vi "uTTA_Calibration_Curr.vi"(6 "AR488_In":refnum<visa-resource-name>, 7 "CommandQueue":refnum<queue>, 8 "error in":errorcluster, 9 "FunctionGen_In":refnum<visa-resource-name>, 10 "DataQueue":refnum<queue>, 11 "TDMS_FileIn":refnum<k34>) -> (0 "error out":errorcluster, 1 "FunctionGen_Out":refnum<visa-resource-name>, 3 "TDMS_FileOut":refnum<k34>, 4 "AR488_Out":refnum<visa-resource-name>)   [LabVIEW 2021]
uses:
  <vilib>/Utility/miscctls.llb/LVPointTypeDef.ctl
  <vilib>/Analysis/6fits.llb/Curve Fitting Criteria.ctl
  <vilib>/Analysis/NI_AALPro.lvlib
panel:
  out "ADC offset":dbl format="%#_6pA"
  out "ADC lin. res":dbl caption="Residue" format="%.3p"
  out "ADC slope":dbl format="%#_4pA/Digit"
  out "ADC_Variance":dbl[](array[numeric]) format="%#.2g"
  out "ADC_Values":dbl[](array[numeric]) format="%#.2g"
  out "Curr ADC Cal.":cluster{"X":dbl, "Y":dbl}[](graph)
  in  "Get Measurement":bool
  in  "Shunt Resistance":dbl=0.00375 format="%#_3pOhm"
  out "Total Measurements":u32
  in  "Complete Cal":bool
  out "Status":string="Exit"
  in  "abort":bool
  # "1. Connect a power supply through a low resistance value shunt ( 10-100mOhm) to the JUT Current Input (J107) of uTTA.\n2. Connect the ground of the power supply to J106 of uTTA.\n3. Connect the sense leads of your multimeter to the sense terminals of the shunt.\n4. Set the power supply to a low current setting (~100mA).\n5. Get a measurement\n6. Set a higher current to the power supply. Steps of 1A to 2A should be sufficient.\n7. Repeat steps 5 and 6 multiple times until you have a good number of measurements.\n8. To finalize the calibration press \"Complete Calibration\"."
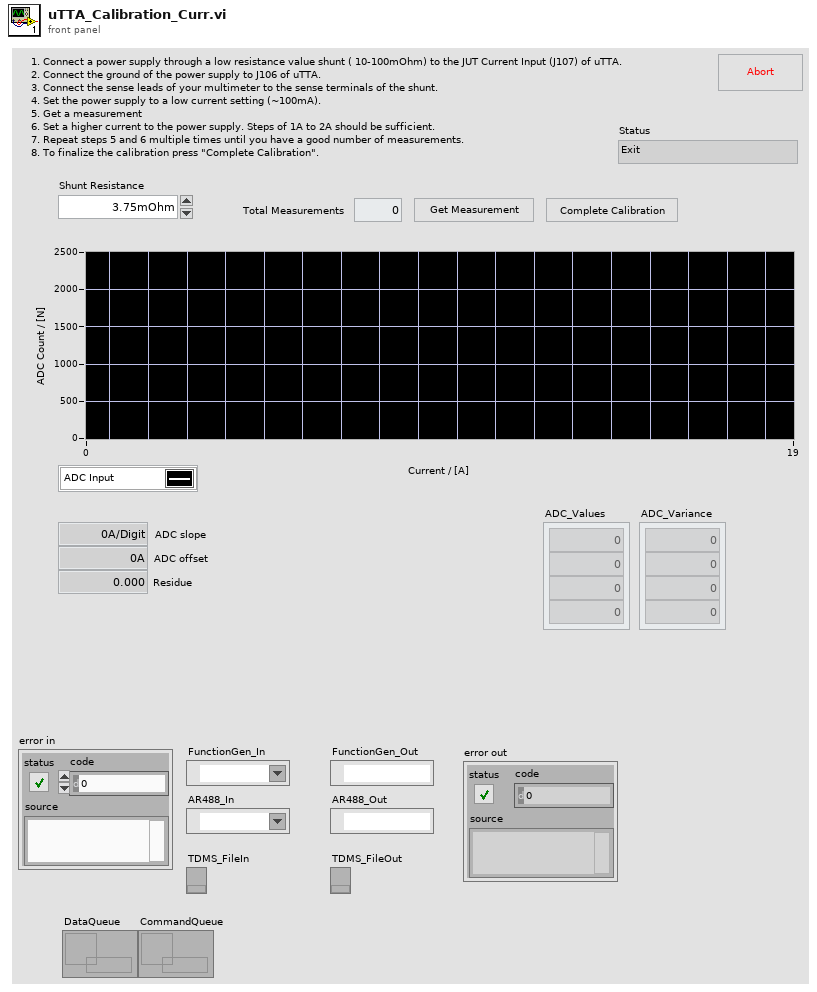
[diagram p1: front panel]
types:
  T1 = typedef "LVPointTypeDef.ctl" = cluster{"Horizontal":i16, "Vertical":i16}
  T2 = enum8{"Enabled", "Disabled", "Disabled and Grayed Out"}
  T3 = typedef "NI_AALPro.lvlib/Curve Fitting Criteria.ctl" = u16
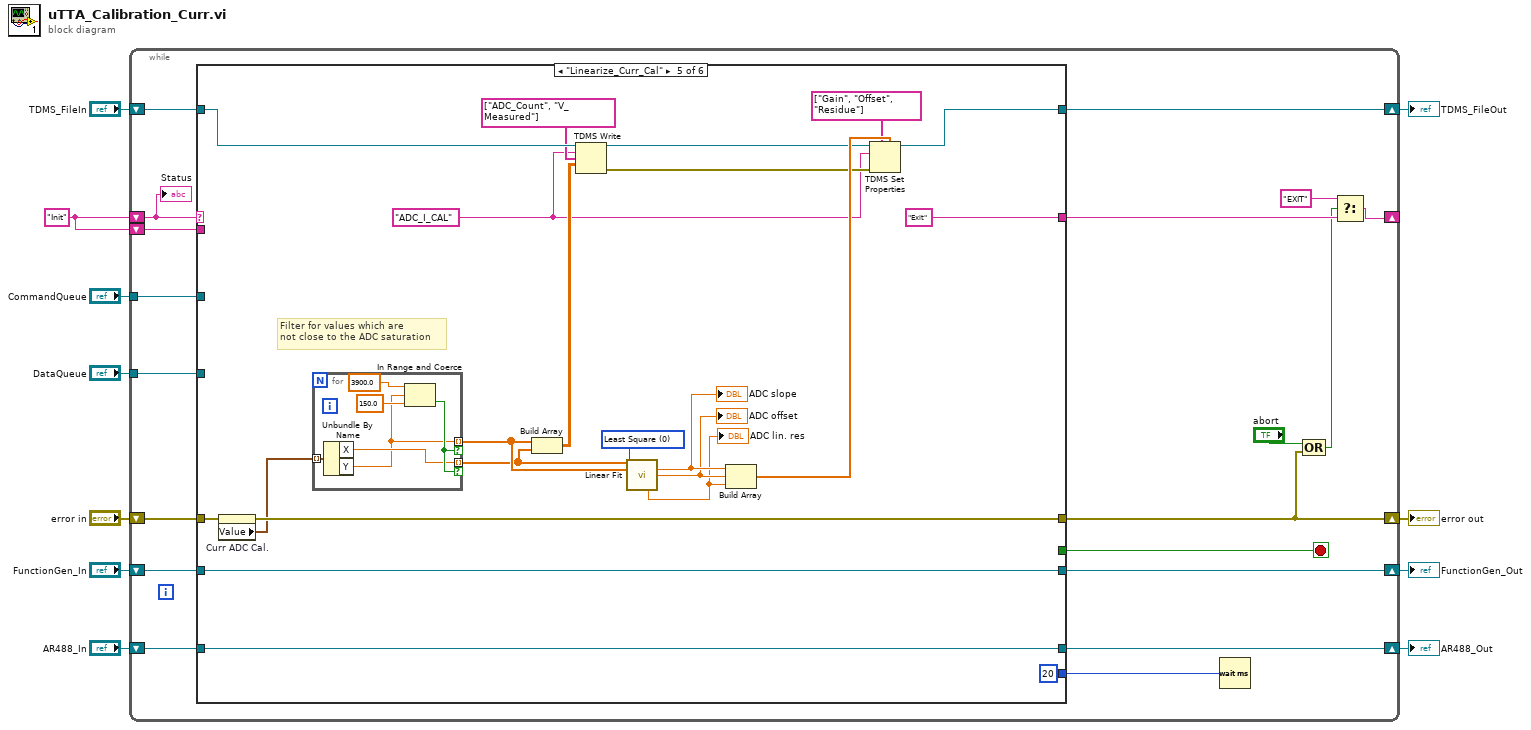
[diagram p0: block diagram]
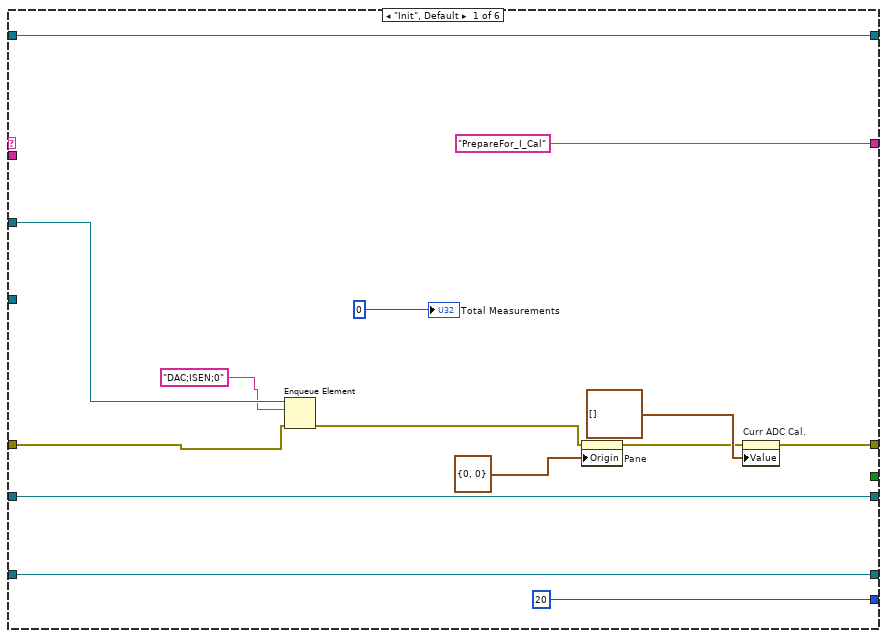
[diagram p2: hidden frame]
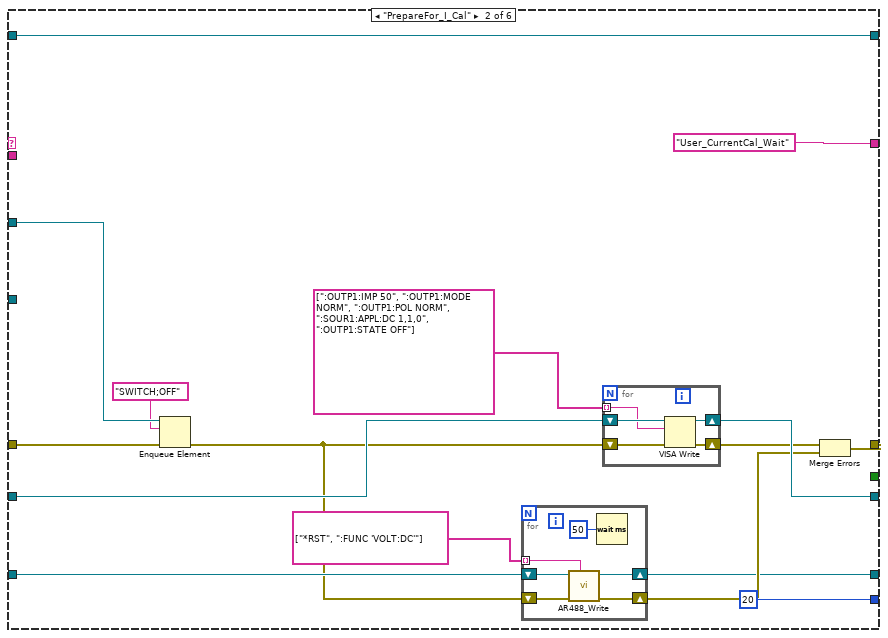
[diagram p3: hidden frame]
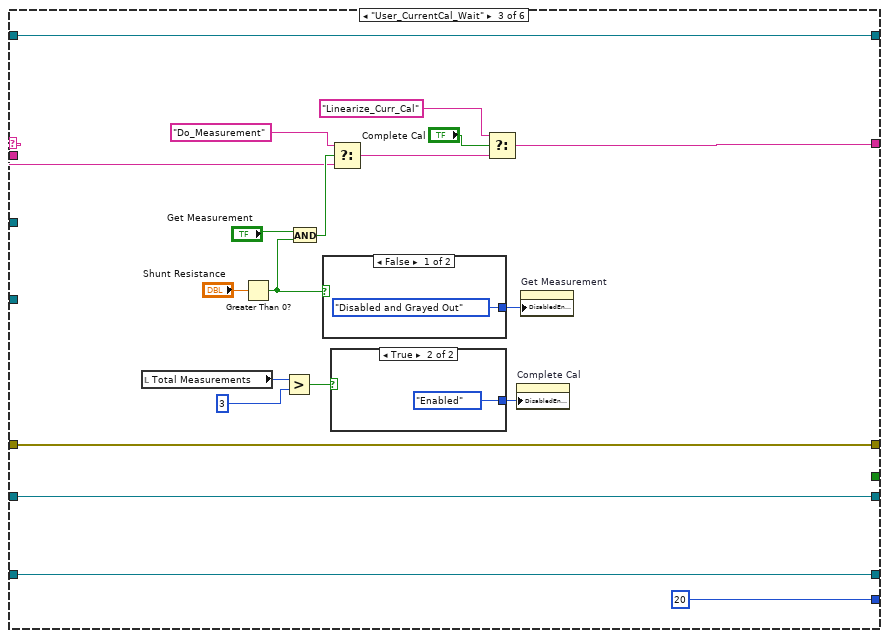
[diagram p4: hidden frame]
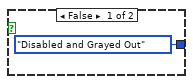
[diagram p5: hidden frame]
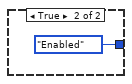
[diagram p6: hidden frame]
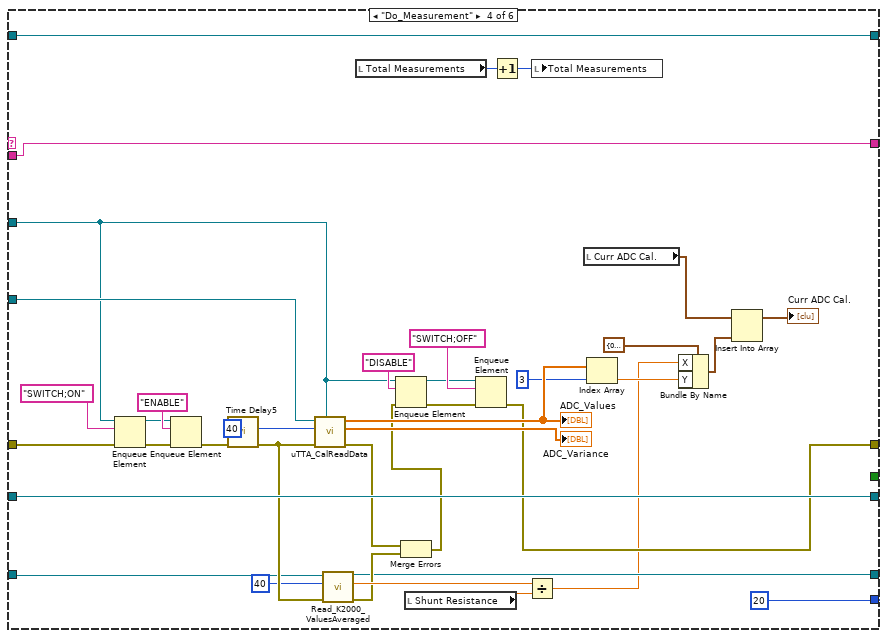
[diagram p7: hidden frame]
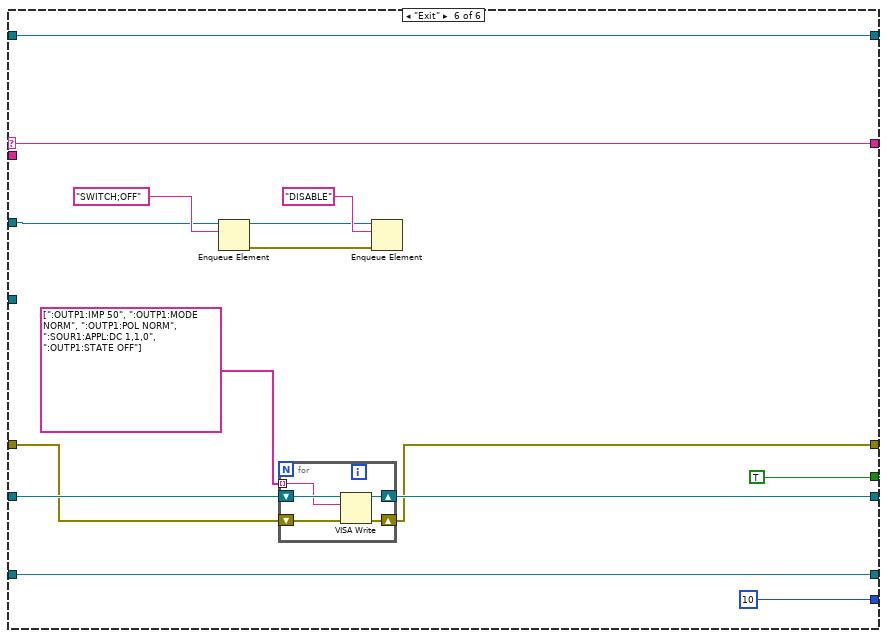
[diagram p8: hidden frame]
diagram:
  w11 = "Init"
  n1 = while {
    shift-right: [w19] -> _
    shift-left: w11 -> [w28]
    shift-right: [w12] -> w2
    shift-left: "error in" -> [w30]
    shift-right: [w26] -> w3
    shift-left: "FunctionGen_In" -> [w27]
    shift-right: [w25] -> w4
    shift-left: "AR488_In" -> [w24]
    shift-left: w11 -> [w23]
    tunnel: "CommandQueue" -> [w22]
    tunnel: "DataQueue" -> [w21]
    shift-right: [w14] -> w1
    shift-left: "TDMS_FileIn" -> [w13]
    stop <- w15 stop-if-true
    n2 = case shown="\"Linearize_Curr_Cal\"" w28 {
      selector: w28 -> [_ _ w73 _ _ w176]
      tunnel: [_ _ _ _ _ TRUE] -> w15
      tunnel: w30 -> [w33 w48 w91 w114 w136 w169]
      tunnel: ["PrepareFor_I_Cal" ("t") "User_CurrentCal_Wait" ("t") w72 w131 "Exit" ("t") w176] -> w20
      tunnel: [w35 w57 w91 w111 w135 w166] -> w12
      tunnel: [u32 20 u32 20 u32 20 u32 20 u32 20 u32 10] -> w29
      tunnel: w27 -> [w41 w50 w90 w133 w154 w171]
      tunnel: [w41 w59 w90 w133 w154 w170] -> w26
      tunnel: [w40 w53 w89 w117 w152 w173] -> w25
      tunnel: w24 -> [w40 w52 w89 w116 w152 w173]
      tunnel: w23 -> [_ _ _ w131 _ _]
      tunnel: w22 -> [w34 w49 _ w97 _ w164]
      tunnel: w21 -> [_ _ _ w115 _ _]
      tunnel: [w39 w51 w88 w132 w150 w168] -> w14
      tunnel: w13 -> [w39 w51 w88 w132 w151 w168]
      frame "Init", Default {
        n3 = Enqueue Element(queue=w34, element="DAC;ISEN;0", error in (no error)=w33) -> (error out=w32:errorcluster)  [unwired: 1 in, 2 out]
        n4 = property on="Pane" class="Pane"(error in=w32, "Origin"=T1 {"Horizontal"=0, "Vertical"=0}) -> (error out=w36:errorcluster)  [unwired: 1 in, 1 out]
        n5 = property on="Curr ADC Cal." class="XYGraph (strict)"(error in=w36, "Value"=cluster{"Voltage mean":dbl, "mean":dbl}[] [] ("History Data")) -> (error out=w35:errorcluster)  [unwired: 1 in, 1 out]
        "Total Measurements" <- u32 0 ("Total Measurements")
      }
      frame "PrepareFor_I_Cal" {
        n6 = Enqueue Element(queue=w49, element="SWITCH;OFF", error in (no error)=w48) -> (error out=w45:errorcluster)  [unwired: 1 in, 2 out]
        n7 = for {
          tunnel: string[] ["*RST", ":FUNC 'VOLT:DC'"] -> [w65] mode=indexing
          shift-right: [w63] -> w53
          shift-left: w52 -> [w66]
          shift-right: [w62] -> w54
          shift-left: w45 -> [w64]
          n8 = call "AR488_Write.vi"("write"=w65, "error in (no error)"=w64, "VISA Refnum in"=w66) -> ("error out"=w62:errorcluster, "VISA Refnum out"=w63:refnum<visa-resource-name>)  [unwired: 7 in]
          n9 = Wait (ms)(milliseconds to wait=u32 50) -> ()  [unwired: 1 out]
        }
        n10 = for {
          shift-right: [w70] -> w59
          shift-left: w50 -> [w71]
          tunnel: string[] [":OUTP1:IMP 50", ":OUTP1:MODE NORM", ":OUTP1:POL NORM", ":SOUR1:APPL:DC 1,1,0", ":OUTP1:STATE OFF"] ("Array 2") -> [w69] mode=indexing
          shift-right: [w67] -> w58
          shift-left: w45 -> [w68]
          n11 = VISA Write(VISA resource name=w71, write buffer=w69, error in (no error)=w68) -> (VISA resource name out=w70:refnum<visa-resource-name>, error out=w67:errorcluster)  [unwired: 1 out]
        }
        n12 = Merge Errors(w58, w54) -> (w57:errorcluster)
      }
      frame "User_CurrentCal_Wait" {
        n13 = local read "Total Measurements"() -> (w84:u32)
        n14 = Greater Than 0?(x="Shunt Resistance") -> (x > 0?=w83:bool)
        n15 = Greater?(x=w84, y=u32 3) -> (0:w85:bool)
        n16 = And(x="Get Measurement", y=w83) -> (x .and. y?=w82:bool)
        n17 = case shown="False" w83 {
          tunnel: [T2."Disabled and Grayed Out" ("Disabled") T2."Enabled" ("Disabled")] -> w75
          frame False {
          }
          frame True {
          }
        }
        n18 = case shown="True" w85 {
          tunnel: [T2."Disabled and Grayed Out" ("Disabled") T2."Enabled" ("Disabled")] -> w74
          frame False {
          }
          frame True {
          }
        }
        n19 = Select(t="Do_Measurement", s=w82, f=w73) -> (s? t:f=w86:string)
        n20 = Select(t="Linearize_Curr_Cal", s="Complete Cal", f=w86) -> (s? t:f=w72:string)
        n21 = property on="Complete Cal" class="Bool"("DisabledEnum"=w74) -> ()  [unwired: 2 in, 2 out]
        n22 = property on="Get Measurement" class="Bool"("DisabledEnum"=w75) -> ()  [unwired: 2 in, 2 out]
      }
      frame "Do_Measurement" {
        n23 = Enqueue Element(queue=w97, element="SWITCH;ON", error in (no error)=w114) -> (queue out=w100:refnum<queue>, error out=w102:errorcluster)  [unwired: 1 in, 1 out]
        n24 = Enqueue Element(queue=w100, element="ENABLE", error in (no error)=w102) -> (error out=w101:errorcluster)  [unwired: 1 in, 2 out]
        n25 = call "Time Delay5"("error in (no error)"=w101) -> ("error out"=w123:errorcluster)  [unwired: 10 in]
        n26 = call "uTTA_CalReadData.vi"("Control Queue"=w97, "error in"=w123, "Averaged Values"=40, "Data Queue in"=w115) -> ("error out"=w124:errorcluster, "ADC_Variance"=→"ADC_Variance":dbl[], "ADC_Values"=w126:dbl[])  [unwired: 3 in, 2 out]
        "ADC_Values" <- w126
        n27 = call "Read_K2000_ValuesAveraged.vi"("error in"=w123, "No. Averaged Values"=40, "VISA Refnum in"=w116) -> ("error out"=w122:errorcluster, "mean"=w128:dbl, "VISA Refnum out"=w117:refnum<visa-resource-name>)  [unwired: 6 in]
        n28 = local read "Total Measurements"() -> (w129:u32)
        n29 = Merge Errors(w124, w122) -> (w99:errorcluster)
        n30 = Enqueue Element(queue=w97, element="DISABLE", error in (no error)=w99) -> (queue out=w96:refnum<queue>, error out=w98:errorcluster)  [unwired: 1 in, 1 out]
        n31 = local read "Shunt Resistance"() -> (w127:dbl)
        n32 = Enqueue Element(queue=w96, element="SWITCH;OFF", error in (no error)=w98) -> (error out=w111:errorcluster)  [unwired: 1 in, 2 out]
        n33 = Increment(x=w129) -> (x+1=w130:u32)
        n34 = Divide(x=w128, y=w127) -> (x/y=w108:dbl)
        n35 = local write "Total Measurements"(w130) -> ()
        n36 = local read "Curr ADC Cal."() -> (w107:cluster{"X":dbl, "Y":dbl}[])
        n37 = Index Array(array=w126, index=3) -> (element=w109:dbl)
        n38 = Bundle By Name(cluster=cluster{"X":dbl, "Y":dbl} {"X"=0.0, "Y"=0.0}, "X"=w108, "Y"=w109) -> (w105:cluster{"X":dbl, "Y":dbl})
        n39 = Insert Into Array(array=w107, new element=w105) -> (→"Curr ADC Cal.":cluster{"X":dbl, "Y":dbl}[])  [unwired: 1 in]
      }
      frame "Linearize_Curr_Cal" {
        w141 = "ADC_I_CAL" ("group name in (Untitled)")
        w155 = T3 0 items=["Least Square", "Least Absolute Residual", "Bisquare"] ("method")
        # "Filter for values which are \nnot close to the ADC saturation"
        n40 = property on="Curr ADC Cal." class="XYGraph (strict)"(error in=w136) -> (error out=w135:errorcluster, "Value"=w134:cluster{"X":dbl, "Y":dbl}[])  [unwired: 1 in, 1 out]
        n41 = for {
          tunnel: w134 -> [w161] mode=indexing
          tunnel: [w157] -> w137 mode=indexing if=w159
          tunnel: [w156] -> w138 mode=indexing if=w159
          n42 = Unbundle By Name(w161) -> ("X"=w157:dbl, "Y"=w156:dbl)
          n43 = In Range and Coerce(upper limit=3900.0, x=w156, lower limit=150.0 ("y")) -> (In Range?=w159:bool)  [unwired: 1 out]
        }
        n44 = Build Array(w138, w137) -> (w149:dbl[][])
        n45 = TDMS Write(0:w151, 5:w141, 7:string[] ["ADC_Count", "V_Measured"], 9:w149) -> (4:w144:refnum<k34>, 15:w143:errorcluster)  [unwired: 2 in, 2 out]
        n46 = call <vilib>:"Linear Fit.vi"("Y"=w137, "X"=w138, "method"=w155) -> ("slope"=w148:dbl, "intercept"=w147:dbl, "residue"=w140:dbl)  [unwired: 8 in, 2 out]
        "ADC offset" <- w147
        "ADC lin. res" <- w140
        "ADC slope" <- w148
        n47 = Build Array(w148, w147, w140) -> (w146:dbl[])
        n48 = TDMS Set Properties(5:w146, 7:string[] ["Gain", "Offset", "Residue"] ("property names"), 8:w143, 10:w141, 11:w144) -> (3:w150:refnum<k34>)  [unwired: 1 in, 3 out]
      }
      frame "Exit" {
        n49 = Enqueue Element(queue=w164, element="SWITCH;OFF") -> (queue out=w163:refnum<queue>, error out=w162:errorcluster)  [unwired: 2 in, 1 out]
        n50 = for {
          shift-right: [w180] -> w170
          shift-left: w171 -> [w181]
          tunnel: string[] [":OUTP1:IMP 50", ":OUTP1:MODE NORM", ":OUTP1:POL NORM", ":SOUR1:APPL:DC 1,1,0", ":OUTP1:STATE OFF"] ("Array 2") -> [w179] mode=indexing
          shift-right: [w177] -> w166
          shift-left: w169 -> [w178]
          n51 = VISA Write(VISA resource name=w181, write buffer=w179, error in (no error)=w178) -> (VISA resource name out=w180:refnum<visa-resource-name>, error out=w177:errorcluster)  [unwired: 1 out]
        }
        n52 = Enqueue Element(queue=w163, element="DISABLE", error in (no error)=w162) -> ()  [unwired: 1 in, 3 out]
      }
    }
    n53 = Wait (ms)(milliseconds to wait=w29) -> ()  [unwired: 1 out]
    n54 = Compound Arithmetic op=OR("abort", w12) -> (w17:bool)
    n55 = Select(t="EXIT", s=w17, f=w20) -> (s? t:f=w19:string)
    "Status" <- w28
  }
  "AR488_Out" <- w4
  "FunctionGen_Out" <- w3
  "error out" <- w2
  "TDMS_FileOut" <- w1
